vi "GUI - Nastran PCH File (V1.00).vi"(5 "error in (no error)":errorcluster, 6 "Application Name":string="GSwForm", 7 "F07 File Path - READ":path, 8 "State Queue":string[](array[string])=["SC: Initialize"]) -> (13 "FRF":T1(array[cluster]), 19 "error out":errorcluster)   [LabVIEW 2020, in "Nastran PCH.lvclass"]
uses:
  Nastran PCH.lvclass
  <vilib>/Utility/sysdir.llb/System Directory Type.ctl
  C:/Users/fcharett/docsWork/coding/20openSourceSPWB/API/Generic Utilities_class/Generic Utilities.lvclass
  <vilib>/addons/_AddQ/G#Object/G#Object.lvclass
  API/Generic Utilities_class/Generic Utilities.lvclass
panel:
  in  "Task":enum32{"Monitor", "Settings"}(tab)
  in  "READ - Select F07 File":bool
  out "State History":string[](array[string])
  out "State Index":i32
  in  "Exit":bool
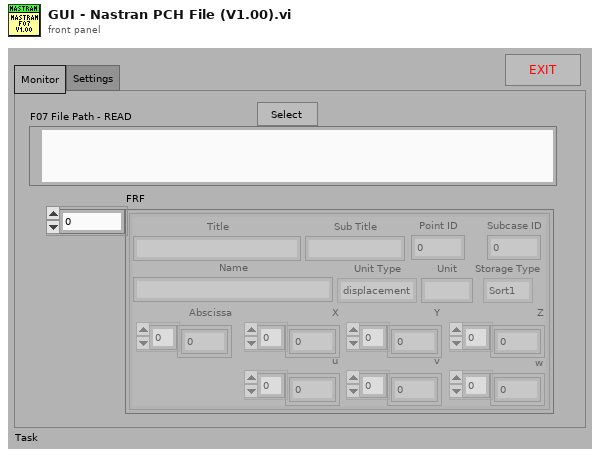
[diagram p1: front panel]
types:
  T1 = cluster{"Title":string, "Sub Title":string, "Point ID":i32, "Subcase ID":i32, "Name":string, "Unit Type":enum16{"displacement", "velocity", "acceleration"}, "Unit":string, "Storage Type":enum16{"Sort1", "Sort2"}, "Abscissa":dbl[], "X":cdb[], "Y":cdb[], "Z":cdb[], "u":cdb[], "v":cdb[], "w":cdb[]}[]
  T2 = enum32{"Invalid", "Standard", "Closed", "Hidden", "Minimized", "Maximized"}
  T3 = typedef "System Directory Type.ctl" = i32
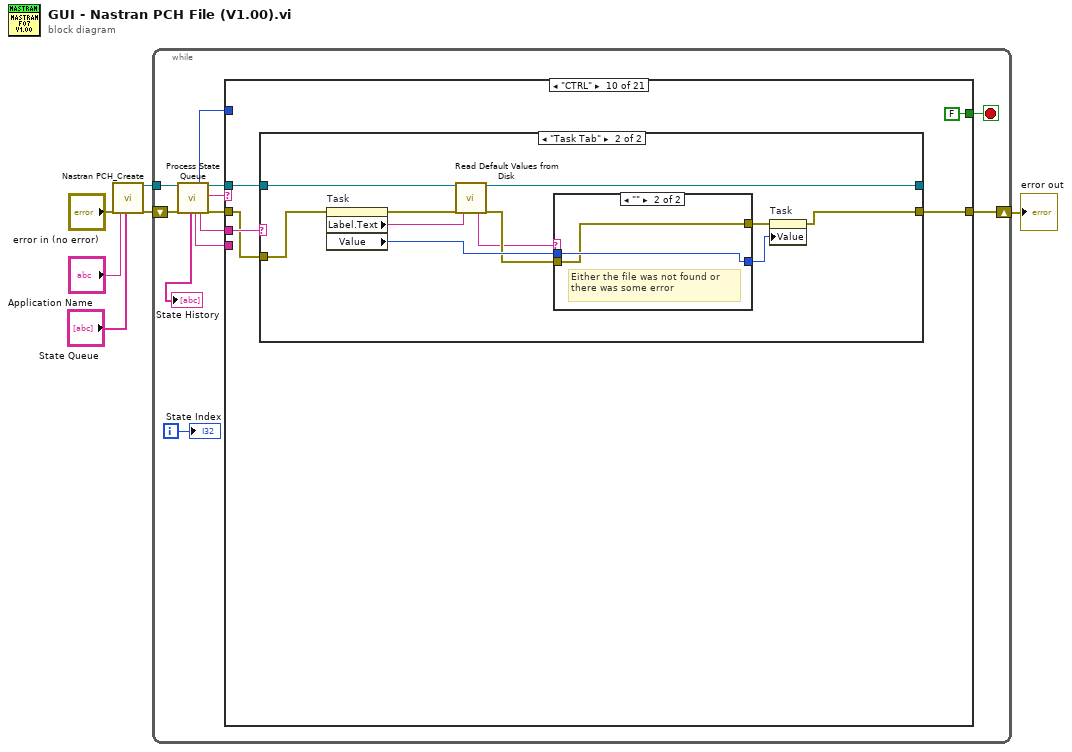
[diagram p0: block diagram]
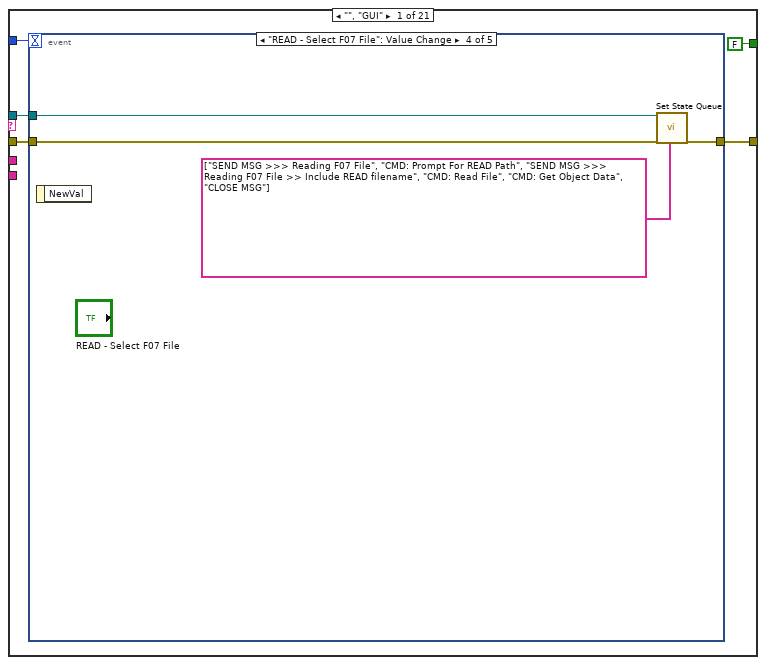
[diagram p2: hidden frame]
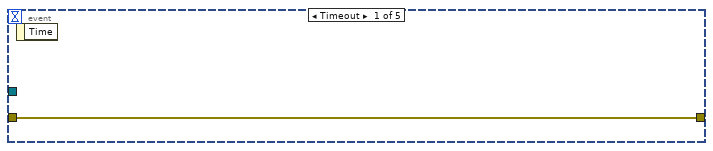
[diagram p3: hidden frame]
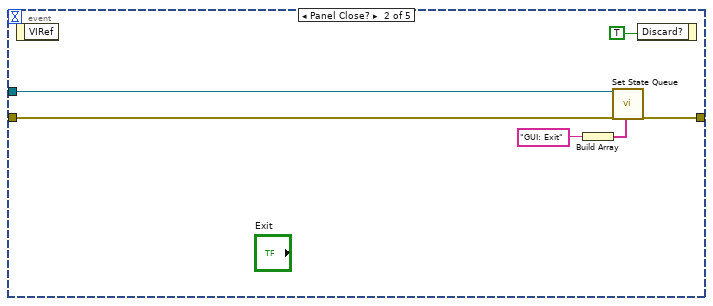
[diagram p4: hidden frame]
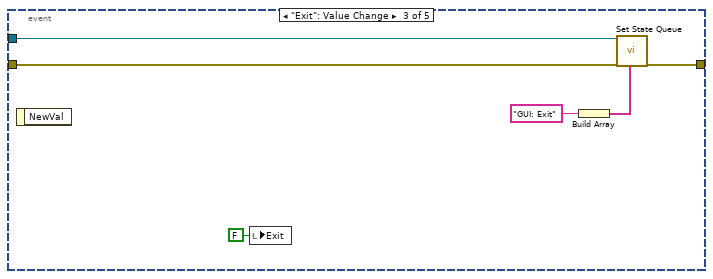
[diagram p5: hidden frame]
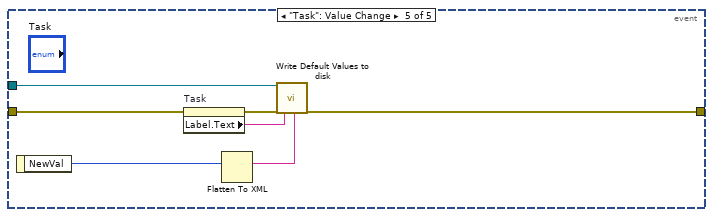
[diagram p6: hidden frame]
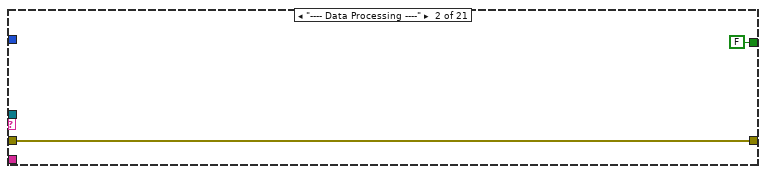
[diagram p7: hidden frame]
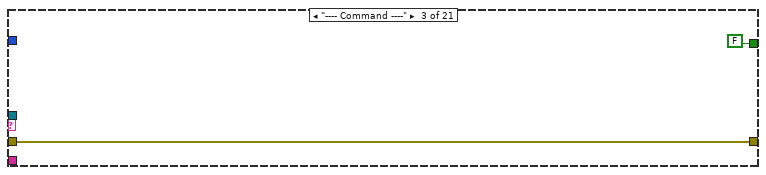
[diagram p8: hidden frame]
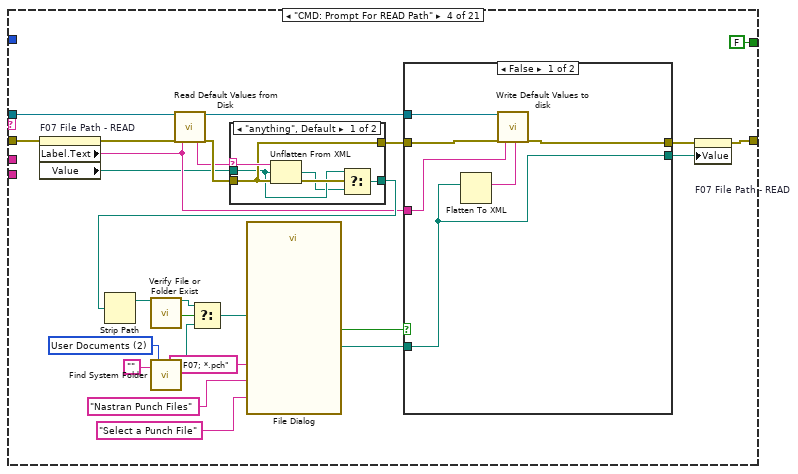
[diagram p9: hidden frame]
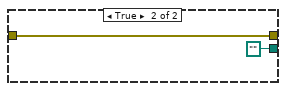
[diagram p10: hidden frame]
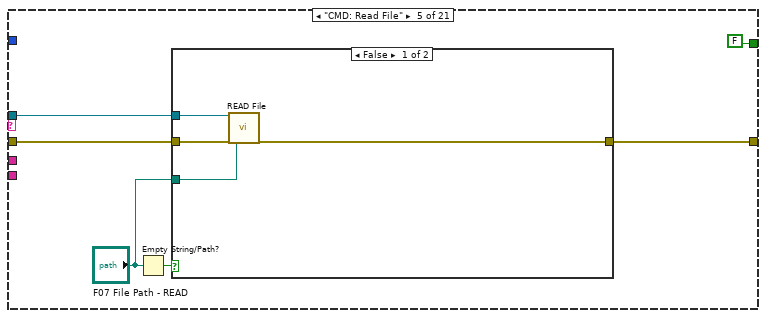
[diagram p12: hidden frame]
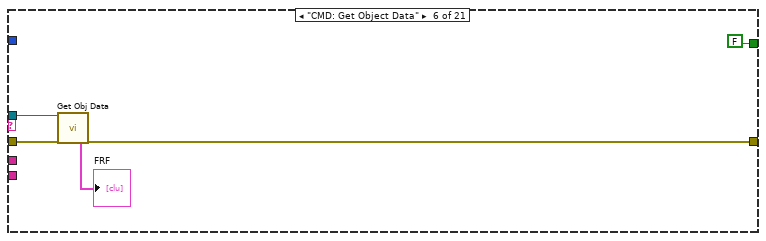
[diagram p14: hidden frame]
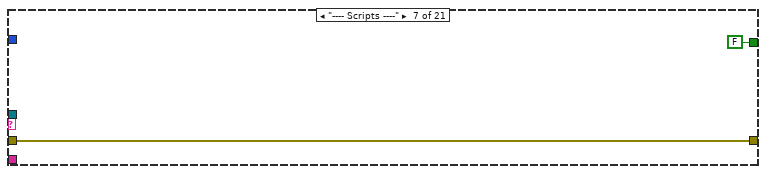
[diagram p15: hidden frame]
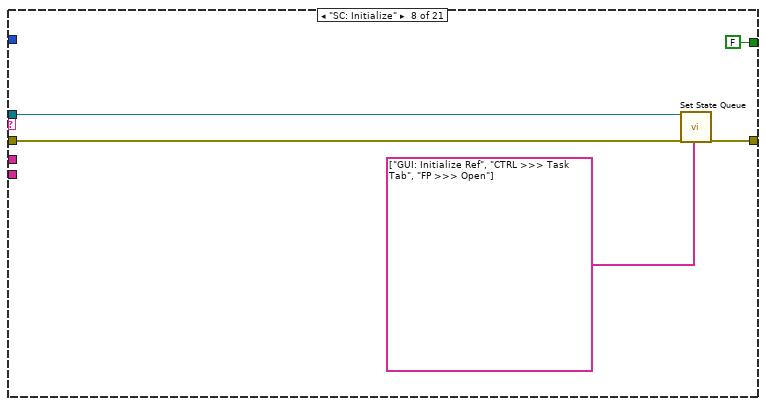
[diagram p16: hidden frame]
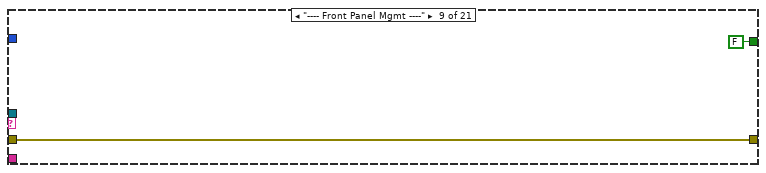
[diagram p17: hidden frame]
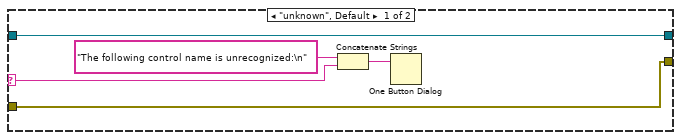
[diagram p18: hidden frame]
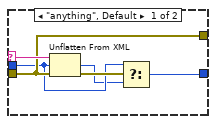
[diagram p19: hidden frame]
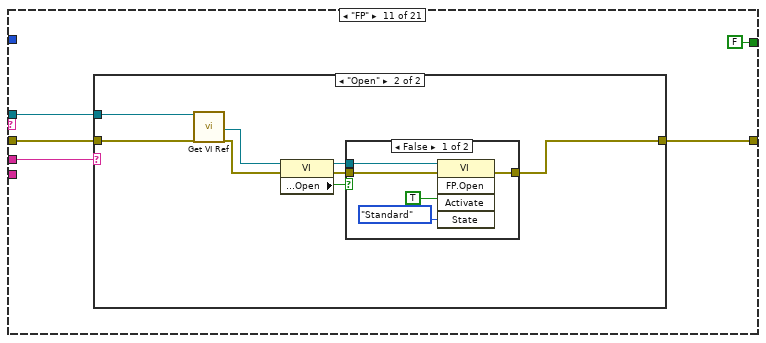
[diagram p20: hidden frame]
diagram:
  n1 = call "Nastran PCH_Create.vi"("error in (no error)"="error in (no error)", "Application Name"="Application Name", "State Queue"="State Queue") -> ("reference out"=w6:refnum<class "Nastran PCH.lvclass">, "error out"=w5:errorcluster)  [unwired: 15 in]
  n2 = while {
    shift-right: [w10] -> w1
    shift-left: w5 -> [w15]
    tunnel: w6 -> [w16]
    i -> [w17]
    stop <- w18 stop-if-true
    n3 = call "Process State Queue.vi"("reference in"=w16, "error in (no error)"=w15) -> ("State History"=→"State History":string[], "Additional Options"=w8:string, "Timeout"=w14:i32, "State Option"=w9:string, "reference out"=w13:refnum<class "Nastran PCH.lvclass">, "Current State"=w12:string, "error out"=w11:errorcluster)  [unwired: 10 in, 1 out]
    n4 = case shown="\"CTRL\"" w12 {
      selector: w12 -> [_ _ _ _ _ _ _ _ _ _ _ _ _ _ _ _ _ w269 _ _ _]
      tunnel: w13 -> [w21 _ _ w53 w94 w106 _ w115 _ w121 w151 _ w180 w187 w221 w251 _ _ _ _ w279]
      tunnel: [FALSE FALSE FALSE FALSE FALSE FALSE FALSE FALSE FALSE FALSE FALSE FALSE FALSE TRUE FALSE FALSE FALSE FALSE FALSE FALSE TRUE] -> w18
      tunnel: w14 -> [w22 _ _ _ _ _ _ _ _ _ _ _ _ _ _ _ _ _ _ _ _]
      tunnel: w9 -> [_ _ _ _ _ _ _ _ _ w122 w148 _ _ _ w230 _ _ _ _ _ _]
      tunnel: w11 -> [w20 w48 w50 w60 w97 w108 w110 w114 w117 w119 w150 w171 w176 w184 w220 w252 w265 w267 w272 w275 w278]
      tunnel: [w19 w48 w50 w55 w96 w105 w110 w113 w117 w120 w149 w171 w177 w183 w218 w248 w265 w267 errorcluster {"status"=FALSE, "code"=0, "source"=""} ("error out") w275 w277] -> w10
      tunnel: w8 -> [_ _ _ _ _ _ _ _ _ _ _ _ _ _ w216 _ _ _ _ _ _]
      frame "", "GUI" {
        n5 = event shown="[3] \"READ - Select F07 File\": Value Change" {
          selector: _ -> [_ _ _ _ _]
          dyn-events: _ -> [_ _ _ _ _]
          timeout: w22 -> [_ _ _ _ _]
          tunnel: w21 -> [_ w28 w34 w39 w46]
          tunnel: w20 -> [w24 w27 w32 w38 w43]
          tunnel: [w24 w26 w33 w40 w41] -> w19
          event Timeout {
            n6 = event-data() -> ()  [unwired: 1 in, 1 out]
          }
          event Panel Close? {
            n7 = event-data() -> ()  [unwired: 1 in, 1 out]
            n8 = Build Array("GUI: Exit") -> (w25:string[])
            n9 = call "Set State Queue.vi"("reference in"=w28, "error in (no error)"=w27, "State Queue"=w25) -> ("error out"=w26:errorcluster)  [unwired: 15 in, 1 out]
            n10 = event-data("Discard?"=TRUE) -> ()  [unwired: 1 in, 1 out]
          }
          event "Exit": Value Change {
            n11 = event-data() -> ()  [unwired: 1 in, 1 out]
            n12 = local write "Exit"(FALSE ("Exit")) -> ()
            n13 = Build Array("GUI: Exit") -> (w31:string[])
            n14 = call "Set State Queue.vi"("reference in"=w34, "error in (no error)"=w32, "State Queue"=w31) -> ("error out"=w33:errorcluster)  [unwired: 15 in, 1 out]
          }
          event "READ - Select F07 File": Value Change {
            n15 = event-data() -> ()  [unwired: 1 in, 1 out]
            n16 = call "Set State Queue.vi"("reference in"=w39, "error in (no error)"=w38, "State Queue"=string[] ["SEND MSG >>> Reading F07 File", "CMD: Prompt For READ Path", "SEND MSG >>> Reading F07 File >> Include READ filename", "CMD: Read File", "CMD: Get Object Data", "CLOSE MSG"]) -> ("error out"=w40:errorcluster)  [unwired: 15 in, 1 out]
          }
          event "Task": Value Change {
            n17 = event-data() -> ("NewVal"=w47:enum32{"Monitor", "Settings"})  [unwired: 1 in]
            n18 = property on="Task" class="TabCtl (strict)"(error in=w43) -> (error out=w42:errorcluster, "Label.Text"=w45:string)  [unwired: 1 in, 1 out]
            n19 = Flatten To XML(6:w47) -> (2:w44:string)
            n20 = call-dynamic "Write Default Values to disk.vi"("reference in"=w46, "error in (no error)"=w42, "Control Label"=w45, "Value (XML String)"=w44) -> ("error out"=w41:errorcluster)  [unwired: 14 in, 1 out]
          }
        }
      }
      frame "---- Data Processing ----" {
      }
      frame "---- Command ----" {
      }
      frame "CMD: Prompt For READ Path" {
        w67 = T3 2 items=["User Home"=0, "User Desktop"=1, "User Documents"=2, "User Application Data"=3, "User Preferences"=4, "User Temporary"=5, "Public Documents"=6, "Public Application Data"=7, "Public Preferences"=8, "Public Cache"=13, "System Core Libraries"=9, "System Installed Libraries"=10, "Application Files"=11, "Boot Volume Root"=12] ("system directory type")
        n21 = property on="F07 File Path - READ" class="Path"(error in=w60) -> (error out=w59:errorcluster, "Label.Text"=w58:string, "Value"=w57:path)  [unwired: 1 in, 1 out]
        n22 = call "Find System Folder.vi"("Application Name"="", "system directory type"=w67) -> ("System Folder"=w68:path)  [unwired: 16 in, 1 out]
        n23 = call-dynamic "Read Default Values from Disk.vi"("reference in"=w53, "error in (no error)"=w59, "Control Label"=w58) -> ("Value (XML String)"=w52:string, "reference out"=w75:refnum<class "Nastran PCH.lvclass">, "error out"=w61:errorcluster)  [unwired: 14 in]
        n24 = case shown="\"anything\", Default" w52 {
          selector: w52 -> [w91 _]
          tunnel: [w86 w93] -> w62
          tunnel: w57 -> [w88 w93]
          tunnel: w61 -> [w89 w92]
          tunnel: [w89 w92] -> w74
          frame "anything", Default {
            n25 = Unflatten From XML(xml string=w91, type=w88, error in (no error)=w89) -> (value=w87:path, error out=w90:errorcluster)
            n26 = Select(t=w88, s=w90, f=w87) -> (s? t:f=w86:path)
          }
          frame "" {
            # "Either the file was not found or there was some error"
          }
        }
        n27 = Strip Path(path=w62) -> (stripped path=w63:path)  [unwired: 1 out]
        n28 = call "Verify File or Folder Exist.vi"("path"=w63) -> ("dup path"=w65:path, "file or folder exists?"=w64:bool)  [unwired: 16 in, 1 out]
        n29 = Select(t=w65, s=w64, f=w68) -> (s? t:f=w66:path)
        n30 = call "File Dialog"("start path"=w66, "button label"="Select a Punch File", "pattern (all files)"="*.F07; *.pch", "pattern label"="Nastran Punch Files") -> ("selected path"=w76:path, "cancelled"=w73:bool)  [unwired: 8 in, 2 out]
        n31 = case shown="False" w73 {
          tunnel: [w79 w85] -> w56
          tunnel: w74 -> [w80 w85]
          tunnel: [w78 path ""] -> w54
          tunnel: w75 -> [w82 _]
          tunnel: w58 -> [w81 _]
          tunnel: w76 -> [w78 _]
          frame False {
            n32 = Flatten To XML(6:w78) -> (2:w83:string)
            n33 = call-dynamic "Write Default Values to disk.vi"("reference in"=w82, "error in (no error)"=w80, "Control Label"=w81, "Value (XML String)"=w83) -> ("error out"=w79:errorcluster)  [unwired: 14 in, 1 out]
          }
          frame True {
          }
        }
        n34 = property on="F07 File Path - READ" class="Path"(error in=w56, "Value"=w54) -> (error out=w55:errorcluster)  [unwired: 1 in, 1 out]
      }
      frame "CMD: Read File" {
        n35 = Empty String/Path?(string/path="F07 File Path - READ") -> (empty?=w98:bool)
        n36 = case shown="False" w98 {
          tunnel: w97 -> [w101 w104]
          tunnel: [w102 w104] -> w96
          tunnel: "F07 File Path - READ" -> [w103 _]
          tunnel: w94 -> [w100 _]
          frame False {
            n37 = call "READ File.vi"("reference in"=w100, "error in (no error)"=w101, "F07 File Path - READ"=w103) -> ("error out"=w102:errorcluster)  [unwired: 15 in, 1 out]
          }
          frame True {
          }
        }
      }
      frame "CMD: Get Object Data" {
        n38 = call "Get Obj Data.vi"("reference in"=w106, "error in (no error)"=w108) -> ("FRF"=→"FRF":T1, "error out"=w105:errorcluster)  [unwired: 15 in, 1 out]
      }
      frame "---- Scripts ----" {
      }
      frame "SC: Initialize" {
        n39 = call "Set State Queue.vi"("reference in"=w115, "error in (no error)"=w114, "State Queue"=string[] ["GUI: Initialize Ref", "CTRL >>> Task Tab", "FP >>> Open"] ("State Queue OUT")) -> ("error out"=w113:errorcluster)  [unwired: 15 in, 1 out]
      }
      frame "---- Front Panel Mgmt ----" {
      }
      frame "CTRL" {
        n40 = case shown="\"Task Tab\"" w122 {
          selector: w122 -> [w127 _]
          tunnel: [w125 w131] -> _
          tunnel: w121 -> [w125 w136]
          tunnel: [w124 w130] -> w120
          tunnel: w119 -> [w124 w134]
          frame "unknown", Default {
            n41 = Concatenate Strings("The following control name is unrecognized:\n", w127) -> (w126:string)
            n42 = One Button Dialog(message=w126) -> ()  [unwired: 1 in, 1 out]
          }
          frame "Task Tab" {
            n43 = property on="Task" class="TabCtl (strict)"(error in=w134) -> (error out=w135:errorcluster, "Label.Text"=w133:string, "Value"=w138:enum32{"Monitor", "Settings"})  [unwired: 1 in, 1 out]
            n44 = call-dynamic "Read Default Values from Disk.vi"("reference in"=w136, "error in (no error)"=w135, "Control Label"=w133) -> ("Value (XML String)"=w129:string, "reference out"=w131:refnum<class "Nastran PCH.lvclass">, "error out"=w132:errorcluster)  [unwired: 14 in]
            n45 = case shown="\"\"" w129 {
              selector: w129 -> [w145 _]
              tunnel: [w140 w147] -> w139
              tunnel: w138 -> [w142 w147]
              tunnel: w132 -> [w143 w146]
              tunnel: [w143 w146] -> w137
              frame "anything", Default {
                n46 = Unflatten From XML(xml string=w145, type=w142, error in (no error)=w143) -> (value=w141:enum32{"Monitor", "Settings"}, error out=w144:errorcluster)
                n47 = Select(t=w142, s=w144, f=w141) -> (s? t:f=w140:enum32{"Monitor", "Settings"})
              }
              frame "" {
                # "Either the file was not found or there was some error"
              }
            }
            n48 = property on="Task" class="TabCtl (strict)"(error in=w137, "Value"=w139) -> (error out=w130:errorcluster)  [unwired: 1 in, 1 out]
          }
        }
      }
      frame "FP" {
        n49 = case shown="\"Open\"" w148 {
          selector: w148 -> [w153 _]
          tunnel: w151 -> [_ w161]
          tunnel: w150 -> [w154 w160]
          tunnel: [w154 w157] -> w149
          frame "unknown", Default {
            n50 = Concatenate Strings("The following FP Command name is unrecognized:\n", w153) -> (w155:string)
            n51 = One Button Dialog(message=w155) -> ()  [unwired: 1 in, 1 out]
          }
          frame "Open" {
            n52 = call-dynamic "Get VI Ref.vi"("reference in"=w161, "error in (no error)"=w160) -> ("GUI VI Ref"=w158:refnum<vi>, "error out"=w159:errorcluster)  [unwired: 14 in, 2 out]
            n53 = property class="VI"(reference=w158, error in=w159) -> (reference out=w163:refnum<vi>, error out=w164:errorcluster, "Front Panel.Open"=w162:bool)
            n54 = case shown="False" w162 {
              tunnel: [w167 w170] -> w157
              tunnel: w164 -> [w166 w170]
              tunnel: w163 -> [w165 _]
              frame False {
                n55 = invoke class="VI" method="FP.Open"(reference=w165, error in=w166, "Activate"=TRUE, "State"=T2."Standard") -> (error out=w167:errorcluster)  [unwired: 1 in, 4 out]
              }
              frame True {
              }
            }
          }
        }
      }
      frame "---- GUI Functions ----" {
      }
      frame "GUI: Initialize Ref" {
        n56 = control-ref of="GUI Reference"() -> (w175:refnum<vi>)
        n57 = call "Set VI Ref.vi"("reference in"=w180, "error in (no error)"=w176, "GUI VI Ref"=w175) -> ("reference out"=w179:refnum<class "Nastran PCH.lvclass">, "error out"=w174:errorcluster)  [unwired: 15 in]
        n58 = call "Set Close Panel (Yes or No).vi"("reference in"=w179, "error in (no error)"=w174) -> ("reference out"=w178:refnum<class "Nastran PCH.lvclass">, "error out"=w173:errorcluster)  [unwired: 16 in]
        n59 = call "Set Message Window Ref.vi"("reference in"=w178, "error in (no error)"=w173) -> ("error out"=w177:errorcluster)  [unwired: 16 in, 1 out]
      }
      frame "GUI: Exit" {
        n60 = call-dynamic "Get Message Window Ref.vi"("reference in"=w187, "error in (no error)"=w184) -> ("reference out"=w186:refnum<class "Nastran PCH.lvclass">, "Msg Win Ref"=w182:refnum<vi>, "error out"=w185:errorcluster)  [unwired: 15 in]
        n61 = call-dynamic "Get VI Ref.vi"("reference in"=w186, "error in (no error)"=w185) -> ("reference out"=w191:refnum<class "Nastran PCH.lvclass">, "GUI VI Ref"=w189:refnum<vi>, "error out"=w190:errorcluster)  [unwired: 14 in, 1 out]
        n62 = call-dynamic "Get Close Panel (Yes or No).vi"("reference in"=w191, "error in (no error)"=w190) -> ("Close Panel?"=w192:bool, "reference out"=w194:refnum<class "Nastran PCH.lvclass">, "error out"=w193:errorcluster)  [unwired: 15 in]
        n63 = call-dynamic "Destroy.vi"("reference in"=w194, "error in (no error)"=w193) -> ("error out"=w198:errorcluster)  [unwired: 16 in, 1 out]
        n64 = call <vilib>:"GarbageCollector.vi"("error in (no error)"=w198) -> ("error out"=w188:errorcluster)  [unwired: 16 in, 2 out]
        n65 = Close Reference(reference=w182, error in (no error)=w188) -> (error out=w197:errorcluster)
        n66 = case shown="True" w192 {
          tunnel: w197 -> [w201 w205]
          tunnel: [w201 w204] -> w195
          tunnel: [w200 w203] -> w196
          tunnel: w189 -> [w200 w202]
          frame False {
          }
          frame True {
            n67 = property class="VI"(reference=w202, error in=w205) -> (reference out=w207:refnum<vi>, error out=w206:errorcluster, "Front Panel.Open"=w208:bool)
            n68 = case shown="True" w208 {
              tunnel: [w210 w214] -> w204
              tunnel: w206 -> [w210 w213]
              tunnel: w207 -> [w209 w212]
              tunnel: [w209 w211] -> w203
              frame False {
              }
              frame True {
                n69 = invoke class="VI" method="FP.Close"(reference=w212, error in=w213) -> (reference out=w211:refnum<vi>, error out=w214:errorcluster)  [unwired: 1 in, 1 out]
              }
            }
          }
        }
        n70 = Close Reference(reference=w196, error in (no error)=w195) -> (error out=w183:errorcluster)
      }
      frame "SEND MSG" {
        n71 = call-dynamic "Get Message Window Ref.vi"("reference in"=w221, "error in (no error)"=w220) -> ("Msg Win Ref"=w217:refnum<vi>, "error out"=w219:errorcluster)  [unwired: 15 in, 1 out]
        n72 = case shown="\"Include READ filename\"" w216 {
          tunnel: ["" w233] -> w215
          frame "None", Default {
          }
          frame "Include READ filename" {
            n73 = local read "F07 File Path - READ"() -> (w236:path)
            n74 = Path To String(path=w236) -> (string=w235:string)
            n75 = Concatenate Strings("\r", w235) -> (w233:string)
          }
        }
        n76 = property class="VI"(reference=w217, error in=w219) -> (reference out=w223:refnum<vi>, error out=w222:errorcluster, "Front Panel.Open"=w224:bool)
        n77 = case shown="False" w224 {
          tunnel: [w243 w247] -> w226
          tunnel: w222 -> [w238 w247]
          tunnel: w223 -> [w240 w246]
          tunnel: [w242 w246] -> w225
          frame False {
            w241 = FALSE ("Wait Until Done")
            n78 = invoke class="VI" method="Run VI"(reference=w240, error in=w238, "Wait until done"=w241, "Auto Dispose Ref"=w241) -> (reference out=w239:refnum<vi>, error out=w237:errorcluster)  [unwired: 1 in, 3 out]
            n79 = invoke class="VI" method="FP.Open"(reference=w239, error in=w237, "Activate"=TRUE, "State"=T2."Standard") -> (reference out=w242:refnum<vi>, error out=w243:errorcluster)  [unwired: 1 in, 3 out]
          }
          frame True {
          }
        }
        n80 = Concatenate Strings("\r\n", w230, w215) -> (w229:string)
        n81 = invoke class="VI" method="Ctrl Val.Set"(reference=w225, error in=w226, "Control Name"="Message", "Value"=w229) -> (error out=w218:errorcluster)  [unwired: 1 in, 4 out]
      }
      frame "CLOSE MSG" {
        n82 = call-dynamic "Get Message Window Ref.vi"("reference in"=w251, "error in (no error)"=w252) -> ("Msg Win Ref"=w249:refnum<vi>, "error out"=w250:errorcluster)  [unwired: 15 in, 1 out]
        n83 = property class="VI"(reference=w249, error in=w250) -> (reference out=w256:refnum<vi>, error out=w257:errorcluster, "Front Panel.Open"=w255:bool)
        n84 = case shown="True" w255 {
          tunnel: [w260 w264] -> w254
          tunnel: w257 -> [w260 w263]
          tunnel: w256 -> [w259 w262]
          tunnel: [w259 w261] -> w253
          frame False {
          }
          frame True {
            n85 = invoke class="VI" method="FP.Close"(reference=w262, error in=w263) -> (reference out=w261:refnum<vi>, error out=w264:errorcluster)  [unwired: 1 in, 1 out]
          }
        }
        n86 = invoke class="VI" method="Abort VI"(reference=w253, error in=w254) -> (error out=w248:errorcluster)  [unwired: 1 in, 2 out]
      }
      frame "---- Miscelleneous ----" {
      }
      frame "unknown", Default {
        n87 = Concatenate Strings("The following state is unrecognized?\n", w269) -> (w268:string)
        n88 = One Button Dialog(message=w268) -> ()  [unwired: 1 in, 1 out]
      }
      frame "Error" {
        n89 = call <vilib>:"General Error Handler.vi"("error in (no error)"=w272) -> ()  [unwired: 10 in, 5 out]
      }
      frame "Next" {
        # "This is an empty case used so the queue does NOT stop if there is an empty string between two valid states!"
      }
      frame "Quit" {
        # "This is the case used to simply exit when this GUI is used as a SubVI!"
        n90 = call-dynamic "Destroy.vi"("reference in"=w279, "error in (no error)"=w278) -> ("error out"=w277:errorcluster)  [unwired: 16 in, 1 out]
      }
    }
    "State Index" <- w17
  }
  "error out" <- w1
